vi "Next Trigger.vi"(1 "Advance Trigger Reset":bool, 2 "Advance Trigger in":bool, 5 "Enable":bool) -> (7 "Advance Trigger received":bool)   [LabVIEW 2014]
panel:
  # "Copyright 2014 Vidrio Technologies\nScanImage 5 software is licensed under the Apache License, Version 2.0 (the \"License\"); you may not use any files contained\nwithin the ScanImage 5 release except in compliance with the License. You may obtain a copy of the License at\n http://www.apache.org/licenses/LICENSE-2.0\nUnless required by applicable law or agreed to in writing, software distributed under the License is distributed on an\n\"AS IS\" BASIS, WITHOUT WARRANTIES OR CONDITIONS OF ANY KIND, either express or implied. See the License for the\n specific language governing permissions and limitations under the License."
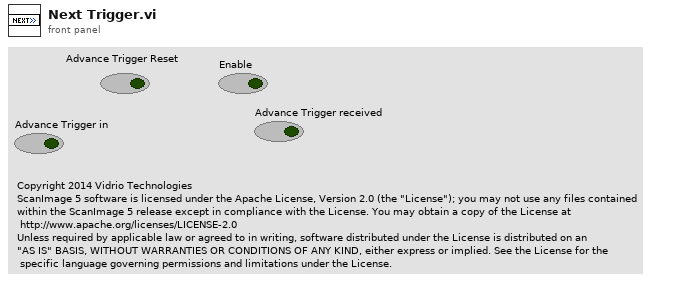
[diagram p1: front panel]
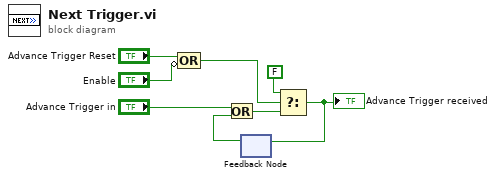
[diagram p0: block diagram]
diagram:
  n1 = Compound Arithmetic op=OR("Advance Trigger Reset", invert "Enable") -> (w1:bool)
  n2 = feedback #1() -> (w6:bool)  [unwired: 1 in]
  n3 = Or(x="Advance Trigger in", y=w6) -> (x .or. y?=w5:bool)
  n4 = Select(t=FALSE ("Advance Trigger received"), s=w1, f=w5) -> (s? t:f=w7:bool)
  "Advance Trigger received" <- w7
  n5 = feedback-in #1(w7) -> ()
